vi "Read Waveform.vi"(8 "error in (no error)":errorcluster, 11 "AOChData in":refnum<class "AOChData.lvclass">) -> (0 "error out":errorcluster, 2 "Waveform":waveform(dbl), 3 "AOChData out":refnum<class "AOChData.lvclass">)   [LabVIEW 2015, in "Analog Output Channel.lvlib" / "AOChData.lvclass"]
uses:
  AOChData.lvclass
  AOChData.lvclass/AOChData.ctl
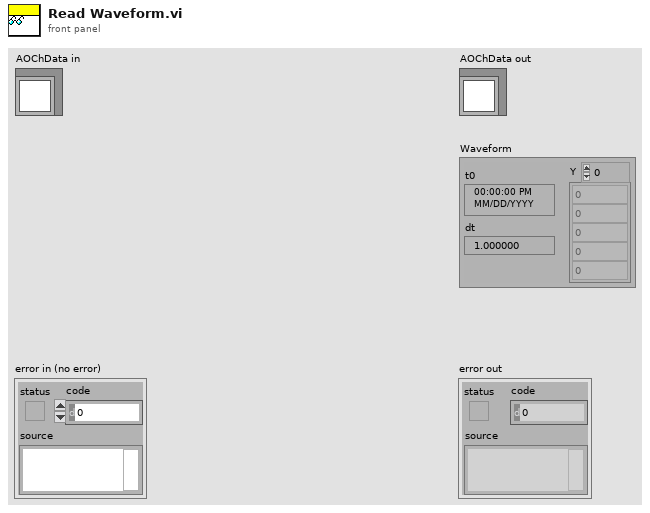
[diagram p1: front panel]
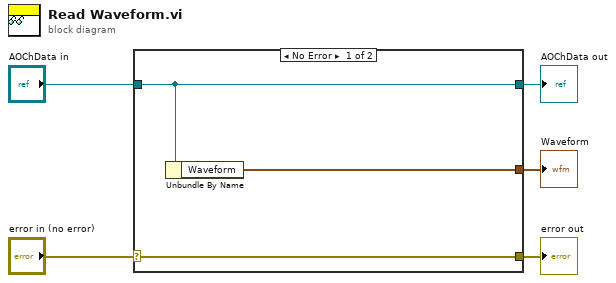
[diagram p0: block diagram]
diagram:
  n1 = case shown="No Error" "error in (no error)" {
    selector: "error in (no error)" -> [w8 w9]
    tunnel: [w8 w9] -> w4
    tunnel: [w7 w10] -> w2
    tunnel: "AOChData in" -> [w7 w10]
    tunnel: [w6 _] -> w1
    frame No Error {
      n2 = Unbundle By Name(w7) -> ("Waveform"=w6:waveform(dbl))
    }
    frame Error {
    }
  }
  "error out" <- w4
  "AOChData out" <- w2
  "Waveform" <- w1
